vi "Alarm UI.vi"(11 "alarms":T3(array[cluster])) -> (2 "UI Alarms":T2[](array[typedef]), 3 "Alarm Model":T1[](array[typedef]) {"Alarm"."value" format="%.2f"; "Alarm"."setpoint" format="%.2f"; "Alarm"."clear time" format="%<%X\n%x>T"; "Alarm"."ack time" format="%<%X\n%x>T"; "Alarm"."set time" format="%<%X\n%x>T"})   [LabVIEW 2018, in "Dynamic Shared Variables.lvlib"]
doc: "Takes the raw Alarm events and creates an Alarm Model and the display to show the alarm ribbon bar."
uses:
  Dynamic Shared Variables.lvlib
  Alarm Cluster (UI).ctl
  Alarm Cluster.ctl
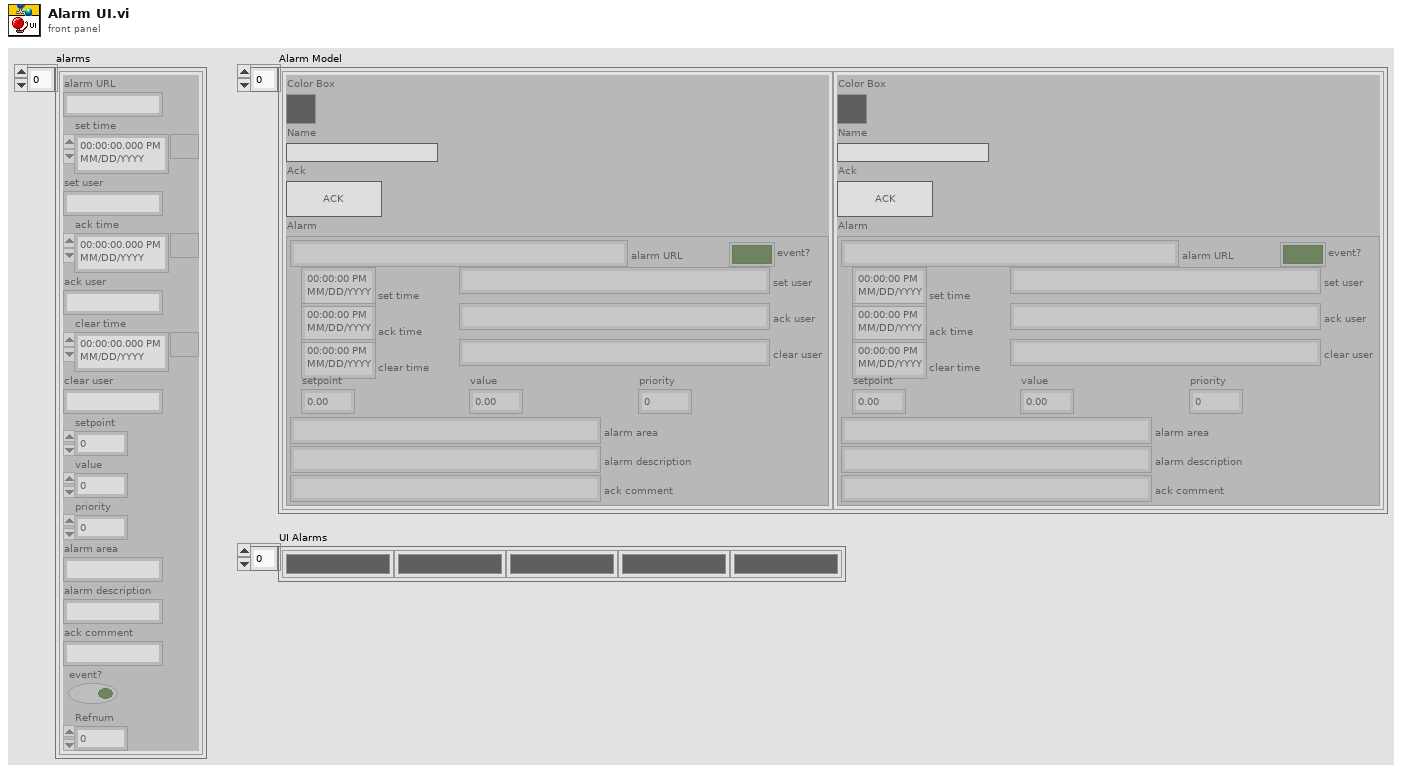
[diagram p1: front panel]
types:
  T1 = typedef "Dynamic Shared Variables.lvlib/Alarm Cluster.ctl" = cluster{"Color Box":u32, "Name":string, "Ack":bool, "Alarm":cluster{"alarm URL":string, "set time":timestamp, "set user":string, "ack time":timestamp, "ack user":string, "clear time":timestamp, "clear user":string, "setpoint":dbl, "value":dbl, "priority":u32, "alarm area":string, "alarm description":string, "ack comment":string, "event?":bool, "Refnum":u64}}
  T2 = typedef "Dynamic Shared Variables.lvlib/Alarm Cluster (UI).ctl" = cluster{"Color Box":u32, "Name":string, "Ack":bool}
  T3 = cluster{"alarm URL":string, "set time":timestamp, "set user":string, "ack time":timestamp, "ack user":string, "clear time":timestamp, "clear user":string, "setpoint":dbl, "value":dbl, "priority":u32, "alarm area":string, "alarm description":string, "ack comment":string, "event?":bool, "Refnum":u64}[]
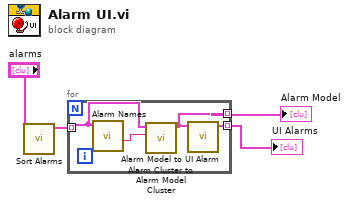
[diagram p0: block diagram]
diagram:
  n1 = call "Sort Alarms.vi"("alarms"="alarms") -> ("alarms out"=w4:T3)  [unwired: 10 in]
  n2 = for {
    tunnel: w4 -> [w7] mode=indexing
    tunnel: [w6] -> w1 mode=indexing
    tunnel: [w5] -> w2 mode=indexing
    n3 = call "Alarm Names.vi"("Alarm"=w7) -> ("Alarm Name"=w8:string)  [unwired: 8 in, 2 out]
    n4 = call "Alarm Cluster to Alarm Model Cluster.vi"("Alarm Name"=w8, "Alarm"=w7) -> ("Alarm Model"=w6:T1)  [unwired: 9 in]
    n5 = call "Alarm Model to UI Alarm.vi"("Alarm Model"=w6) -> ("UI Alarm"=w5:T2)  [unwired: 10 in]
  }
  "UI Alarms" <- w2
  "Alarm Model" <- w1
